vi "Suppress Error Code - Scalar.vi"(8 "Error In":errorcluster, 9 "Error Code":i32) -> (0 "Error Out":errorcluster, 1 "Error Supressed?":bool)   [LabVIEW 2015]
doc: "Clears the specific error passed in, but leaves any other untouched.\n\nFreeware from Moore Good Ideas, www.mooregoodideas.com. Do not remove this line."
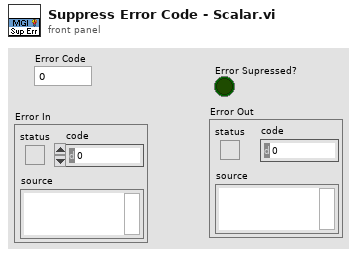
[diagram p1: front panel]
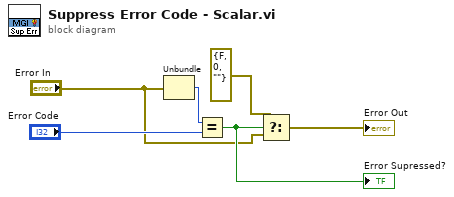
[diagram p0: block diagram]
diagram:
  n1 = Unbundle("Error In") -> ("code"=w3:i32)  [unwired: 2 out]
  n2 = Equal?(x=w3, y="Error Code") -> (x = y?=w5:bool)
  "Error Supressed?" <- w5
  n3 = Select(t=errorcluster {"status"=FALSE, "code"=0, "source"=""} ("error IO"), s=w5, f="Error In") -> (s? t:f=→"Error Out":errorcluster)
